vi "Draw Selection.vi"(0 "Display State In":T1={"Nspeakers"=0, "actions"=[], "Wspeaker"=0, "Wmic"=0, "sel mic"=0, "hover"={"type"=enum."None", "index"=0}, "locked"=FALSE, "states"=[], "sel speak"=13, "selected"=refnum, "Events"={"Mic change"=refnum, "Selection change"=refnum}}, 5 "Layout":T6) -> (4 "empty picture":picture, 8 "String":string)   [LabVIEW 2015, in "HRTF Config.xctl"]
uses:
  HRTF Config.xctl
  Item.ctl
  Layout.ctl
  Hover Item.ctl
  Hover Data.ctl
  State.vi
  Speaker State.ctl
  Events.ctl
  Selection changed.ctl
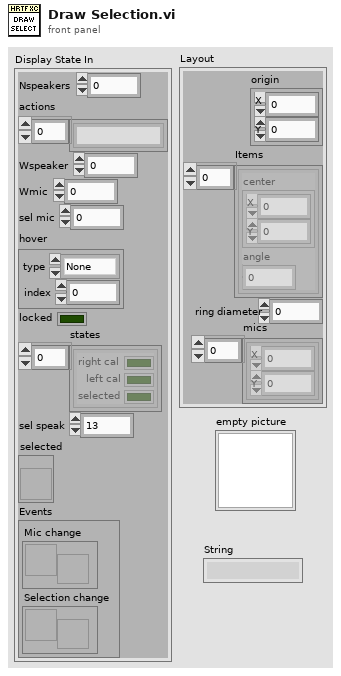
[diagram p1: front panel]
types:
  T1 = typedef "HRTF Config.xctl/State.vi" = cluster{"Nspeakers":i32, "actions":string[], "Wspeaker":i32, "Wmic":i32, "sel mic":i32, "hover":T2, "locked":bool, "states":T4[], "sel speak":i32, "selected":refnum<vi>, "Events":T5}
  T2 = typedef "HRTF Config.xctl/Hover Data.ctl" = cluster{"type":T3, "index":i32}
  T3 = typedef "HRTF Config.xctl/Hover Item.ctl" = enum16{"None", "Speaker", "Mic"}
  T4 = typedef "HRTF Config.xctl/Speaker State.ctl" = cluster{"right cal":bool, "left cal":bool, "selected":bool}
  T5 = typedef "HRTF Config.xctl/Events.ctl" = cluster{"Mic change":refnum<user-event>, "Selection change":refnum<user-event>}
  T6 = typedef "HRTF Config.xctl/Layout.ctl" = cluster{"origin":cluster{"X":i32, "Y":i32}, "Items":T7[], "ring diameter":i32, "mics":cluster{"X":i32, "Y":i32}[]}
  T7 = typedef "HRTF Config.xctl/Item.ctl" = cluster{"center":cluster{"X":i32, "Y":i32}, "angle":dbl}
  T8 = cluster{"Width":i16, "Style":enum32{"Solid", "Dash", "Dot", "DashDot", "DashDotDot"}}
  T9 = cluster{"left":i16, "top":i16, "right":i16, "bottom":i16}
  T10 = cluster{"left":i32, "top":i32, "right":i32, "bottom":i32}
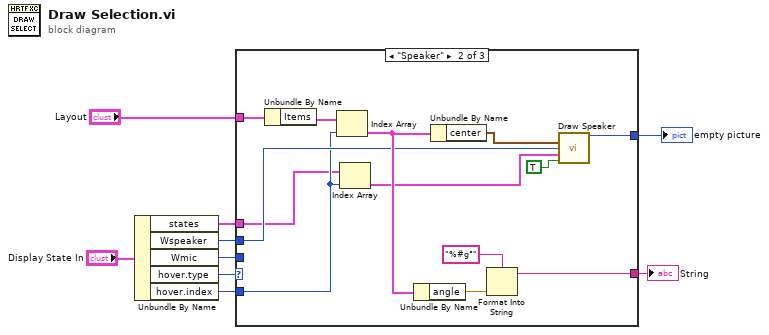
[diagram p0: block diagram]
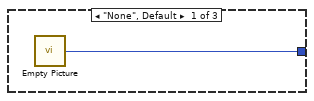
[diagram p2: hidden frame]
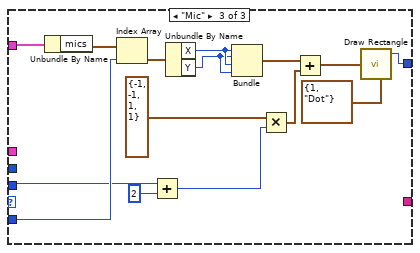
[diagram p3: hidden frame]
diagram:
  n1 = Unbundle By Name("Display State In") -> ("states"=w1:T4[], "Wspeaker"=w3:i32, "Wmic"=w5:i32, "hover.type"=w6:T3, "hover.index"=w4:i32)
  n2 = case shown="\"Speaker\"" w6 {
    tunnel: "Layout" -> [_ w23 w38]
    tunnel: [w10 w18 w25] -> w9
    tunnel: w5 -> [_ _ w29]
    tunnel: w4 -> [_ w14 w36]
    tunnel: w3 -> [_ w15 _]
    tunnel: [_ w19 _] -> w2
    tunnel: w1 -> [_ w13 _]
    frame "None", Default {
      n3 = call "Empty Picture"() -> ("empty picture"=w10:picture)
    }
    frame "Speaker" {
      n4 = Unbundle By Name(w23) -> ("Items"=w22:T7[])
      n5 = Index Array(array=w22, index=w14) -> (element=w17:T7)
      n6 = Index Array(array=w13, index=w14) -> (element=w12:T4)
      n7 = Unbundle By Name(w17) -> ("angle"=w21:dbl)
      n8 = Unbundle By Name(w17) -> ("center"=w16:cluster{"X":i32, "Y":i32})
      n9 = Format Into String(format string="%#g°", w21) -> (resulting string=w19:string)  [unwired: 2 in, 1 out]
      n10 = call "Draw Speaker.vi"("center"=w16, "width"=w15, "state"=w12, "active"=TRUE) -> ("picture out"=w18:picture)  [unwired: 11 in]
    }
    frame "Mic" {
      n11 = Unbundle By Name(w38) -> ("mics"=w37:cluster{"X":i32, "Y":i32}[])
      n12 = Index Array(array=w37, index=w36) -> (element=w30:cluster{"X":i32, "Y":i32})
      n13 = Add(x=w29, y=2) -> (x+y=w27:i32)
      n14 = Unbundle By Name(w30) -> ("X"=w33:i32, "Y"=w32:i32)
      n15 = Bundle("X"=w33, "Y"=w32, "X"=w33, "Y"=w32) -> (w34:cluster{"X":i32, "Y":i32, "X":i32, "Y":i32})  [unwired: 1 in]
      n16 = Multiply(x=T9 {"left"=-1, "top"=-1, "right"=1, "bottom"=1} ("rect"), y=w27) -> (x*y=w35:T10)
      n17 = Add(x=w34, y=w35) -> (x+y=w26:cluster{i32, i32, i32, i32})
      n18 = call <vilib>:"Draw Rectangle.vi"("rect"=w26, "pen"=T8 {"Width"=1, "Style"=enum."Dot"}) -> ("new picture"=w25:picture)  [unwired: 7 in]
    }
  }
  "empty picture" <- w9
  "String" <- w2
